vi "ActionVIOnCompile.vi"(8 "error in (no error)":errorcluster, 11 "Device Item Ref in":T1 format="%.0x") -> (0 "error out":errorcluster)   [LabVIEW 2024, in "Nominal Client System Explorer.lvlib"]
uses:
  Nominal Client System Explorer.lvlib
  <vilib>/NI VeriStand/Custom Device API/Custom Device Item Ref.ctl
  Shared/Compiled.Settings.ctl
  <vilib>/NI VeriStand/Custom Device API/Get Item Property (U16).vi
  <vilib>/NI VeriStand/Custom Device API/Set Item Property (Variant).vi
  <vilib>/NI VeriStand/Custom Device Tools/Custom Device Utility Library/Custom Device Utility Library.lvlib
  <vilib>/NI VeriStand/Custom Device Tools/Custom Device Utility Library/NI VeriStand - Search for Item by Name.vi
  <vilib>/NI VeriStand/Custom Device API/Custom Device API.lvlib
  <vilib>/NI/NIVS Inline Async API/_Data Access System Explorer/Data Access System Explorer.lvlib
  Shared/Nominal Client Shared.lvlib
  Scripting/Nominal Client Scripting.lvlib
  Built/Nominal Client/Windows/nominal-labview-client.lvlibp
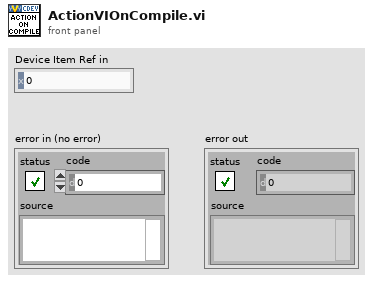
[diagram p1: front panel]
types:
  T1 = typedef "Custom Device API.lvlib/Custom Device Item Ref.ctl" = u64
  T2 = cluster{"Name":string, "Type":enum16{"Output/Write", "Input/Read", "Input/ReadWrite"}, "VS Refs":T1[]}
  T3 = enum16{"Output/Write", "Input/Read", "Input/ReadWrite"}
  T4 = enum16{"open", "replace", "create", "open or create", "replace or create", "replace or create with confirmation"}
  T5 = typedef "Nominal Client Shared.lvlib/Compiled.Settings.ctl" = cluster{"Name":string, "Async Init Timeout":u16, "api key":string}
  T6 = typedef "Custom Device API.lvlib/Custom Device Item Info.ctl" = cluster{"Name":string, "Is Channel":bool, "GUID":string, "Is Waveform":bool}
  T7 = cluster{"Name":string, "Type":enum16{"Output/Write", "Input/Read", "Input/ReadWrite"}, "VS Refs":T1[]}[]
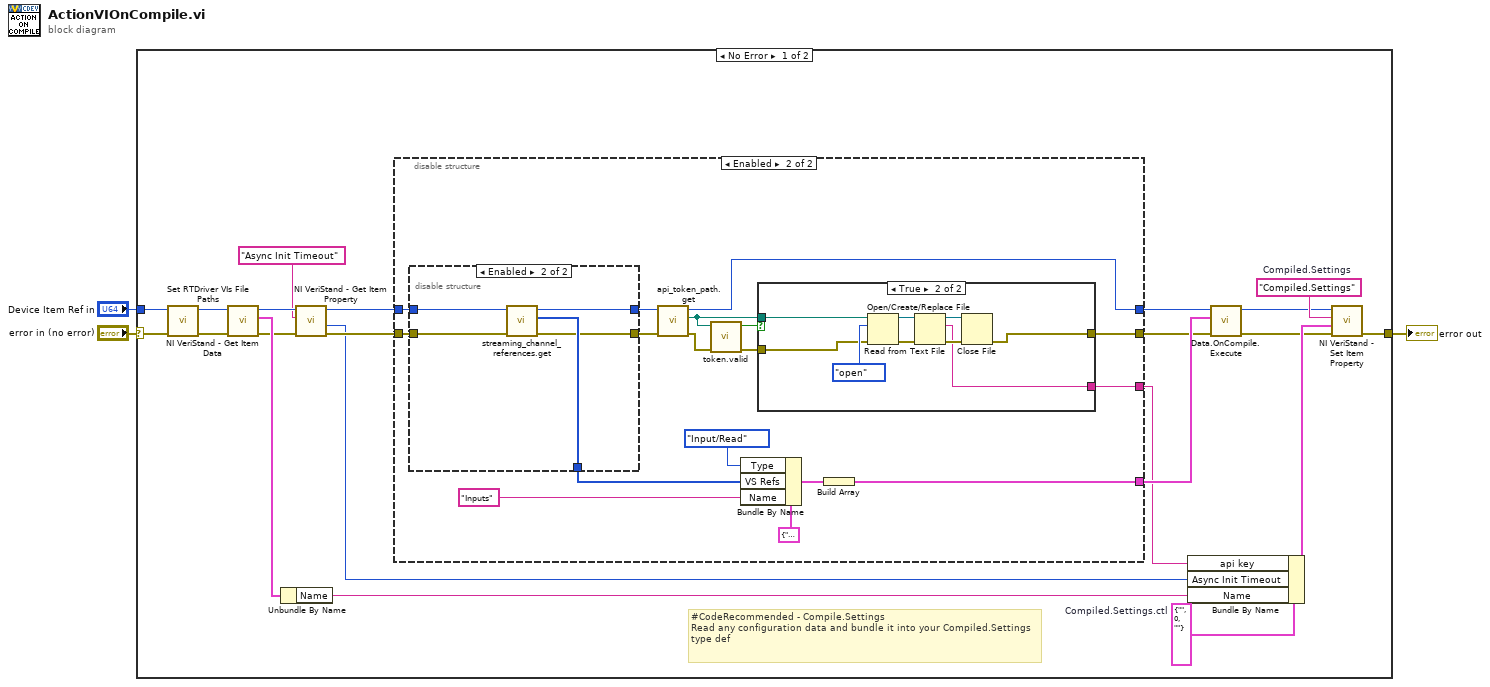
[diagram p0: block diagram]
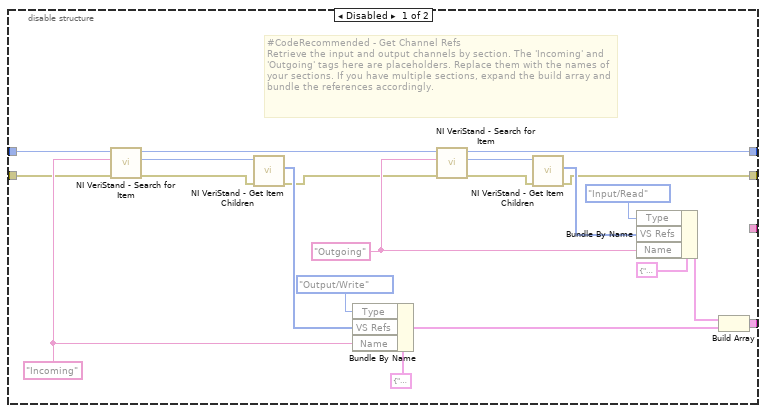
[diagram p2: hidden frame]
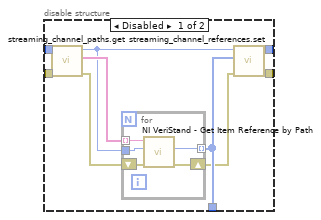
[diagram p3: hidden frame]
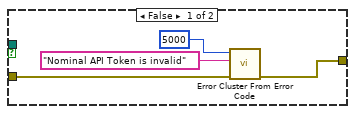
[diagram p4: hidden frame]
diagram:
  n1 = case shown="No Error" "error in (no error)" {
    selector: "error in (no error)" -> [w7 w96]
    tunnel: [w23 w96] -> w2
    tunnel: "Device Item Ref in" -> [w8 _]
    frame No Error {
      w15 = T5 {"Name"="", "Async Init Timeout"=0, "api key"=""}  # Compiled.Settings.ctl
      w25 = "Compiled.Settings"  # Compiled.Settings
      # "#CodeRecommended - Compile.Settings\nRead any configuration data and bundle it into your Compiled.Settings type def"
      n2 = call "Set RTDriver VIs File Paths.vi"("error in (no error)"=w7, "Item Ref in"=w8) -> ("error out"=w5:errorcluster, "Item Ref out"=w6:T1)  [unwired: 8 in]
      n3 = call <vilib>:"NI VeriStand - Get Item Data.vi"("error in (no error)"=w5, "Item Ref in"=w6) -> ("error out"=w14:errorcluster, "Item Info"=w22:T6, "Item Ref out"=w12:T1)  [unwired: 6 in, 1 out]
      n4 = Unbundle By Name(w22) -> ("Name"=w21:string)
      n5 = call-poly <vilib>:"NI VeriStand - Get Item Property.vi"("error in (no error)"=w14, "Property Name"="Async Init Timeout", "Item Ref in"=w12) -> ("error out"=w13:errorcluster, "Value"=w9:u16, "Item Ref out"=w11:T1)  [unwired: 5 in, 1 out]
      n6 = disable-structure shown="Enabled" {
        disable-tunnel: [w37 w59] -> w20
        disable-tunnel: [w33 w57] -> w19
        disable-tunnel: [w32 w58] -> w18
        disable-tunnel: w13 -> [w29 w50]
        disable-tunnel: w11 -> [w28 w51]
        disable-tunnel: [_ w56] -> w4
        frame Disabled {
          w42 = "Outgoing" ("Item Name")
          w44 = "Incoming" ("Item Name")
          # "#CodeRecommended - Get Channel Refs\nRetrieve the input and output channels by section. The 'Incoming' and 'Outgoing' tags here are placeholders. Replace them with the names of your sections. If you have multiple sections, expand the build array and bundle the references accordingly."
          n7 = call-poly <vilib>:"NI VeriStand - Search for Item.vi"("error in"=w29, "Item Name"=w44, "Section Ref in"=w28) -> ("error out"=w27:errorcluster, "Item Ref"=w26:T1, "Section Ref out"=w31:T1)  [unwired: 5 in, 1 out]
          n8 = call <vilib>:"NI VeriStand - Get Item Children.vi"("error in (no error)"=w27, "Item Ref in"=w26) -> ("error out"=w30:errorcluster, "Child Refs"=w43:T1[])  [unwired: 6 in, 2 out]
          n9 = Bundle By Name(cluster=T2 {"Name"="", "Type"=enum."Output/Write", "VS Refs"=[]} ("Group"), "Type"=T3."Output/Write", "VS Refs"=w43, "Name"=w44) -> (w34:T2)
          n10 = call-poly <vilib>:"NI VeriStand - Search for Item.vi"("error in"=w30, "Item Name"=w42, "Section Ref in"=w31) -> ("error out"=w45:errorcluster, "Item Ref"=w46:T1, "Section Ref out"=w32:T1)  [unwired: 5 in, 1 out]
          n11 = call <vilib>:"NI VeriStand - Get Item Children.vi"("error in (no error)"=w45, "Item Ref in"=w46) -> ("error out"=w33:errorcluster, "Child Refs"=w38:T1[])  [unwired: 6 in, 2 out]
          n12 = Bundle By Name(cluster=T2 {"Name"="", "Type"=enum."Output/Write", "VS Refs"=[]} ("Group"), "Type"=T3."Input/Read", "VS Refs"=w38, "Name"=w42) -> (w40:T2)
          n13 = Build Array(w40, w34) -> (w37:T7)
        }
        frame Enabled {
          n14 = disable-structure shown="Enabled" {
            disable-tunnel: w51 -> [w71 w82]
            disable-tunnel: w50 -> [w70 w78]
            disable-tunnel: [w69 w80] -> w49
            disable-tunnel: [w68 w79] -> w48
            disable-tunnel: [w67 w81] -> w47
            frame Disabled {
              n15 = call "streaming_channel_paths.get.vi"("error in (no error)"=w70, "Item Ref in"=w71) -> ("error out"=w65:errorcluster, "Channel Paths"=w72:string[], "Item Ref out"=w66:T1)  [unwired: 7 in]
              n16 = for {
                tunnel: w72 -> [w77] mode=indexing
                tunnel: [w76] -> w67 mode=indexing
                tunnel: w66 -> [w75]
                shift-right: [w74] -> w64
                shift-left: w65 -> [w73]
                n17 = call <vilib>:"NI VeriStand - Get Item Reference by Path.vi"("error in (no error)"=w73, "Root Ref"=w75, "Item Path in"=w77) -> ("error out"=w74:errorcluster, "Item Ref"=w76:T1)  [unwired: 5 in, 2 out]
              }
              n18 = call "streaming_channel_references.set.vi"("error in (no error)"=w64, "Dependent Node Refs"=w67, "Item Ref in"=w66) -> ("error out"=w68:errorcluster, "Item Ref out"=w69:T1)  [unwired: 7 in]
            }
            frame Enabled {
              n19 = call "streaming_channel_references.get.vi"("error in (no error)"=w78, "Item Ref in"=w82) -> ("error out"=w79:errorcluster, "Streaming Channel Refs"=w81:T1[], "Item Ref out"=w80:T1)  [unwired: 7 in]
            }
          }
          n20 = call "api_token_path.get.vi"("error in (no error)"=w48, "Nominal IO Client in"=w49) -> ("error out"=w54:errorcluster, "API Token file"=w55:path, "Nominal IO Client out"=w58:T1)  [unwired: 6 in, 1 out]
          n21 = call "token.valid.vi"("error in"=w54, "token"=w55) -> ("error out"=w53:errorcluster, "valid"=w52:bool)  [unwired: 8 in]
          n22 = Bundle By Name(cluster=T2 {"Name"="", "Type"=enum."Output/Write", "VS Refs"=[]} ("Group"), "Type"=T3."Input/Read", "VS Refs"=w47, "Name"="Inputs") -> (w60:T2)
          n23 = case shown="True" w52 {
            tunnel: [w83 w90] -> w57
            tunnel: [_ w89] -> w56
            tunnel: w55 -> [_ w88]
            tunnel: w53 -> [w84 w87]
            frame False {
              n24 = call <vilib>:"Error Cluster From Error Code.vi"("error in (no error)"=w84, "error message (\"\")"="Nominal API Token is invalid" ("error message (\"\")"), "error code (0)"=5000) -> ("error out"=w83:errorcluster)  [unwired: 6 in]
            }
            frame True {
              n25 = Open/Create/Replace File(file path (use dialog)=w88, error in=w87, operation (0:open)=T4."open") -> (refnum out=w94:refnum<file>, error out=w92:errorcluster)  [unwired: 3 in, 1 out]
              n26 = Read from Text File(file (use dialog)=w94, error in=w92) -> (refnum out=w95:refnum<file>, text=w89:string, error out=w93:errorcluster)  [unwired: 2 in, 1 out]
              n27 = Close File(refnum=w95, error in=w93) -> (error out=w90:errorcluster)  [unwired: 1 out]
            }
          }
          n28 = Build Array(w60) -> (w59:T7)
        }
      }
      n29 = Bundle By Name(cluster=w15, "api key"=w4, "Async Init Timeout"=w9, "Name"=w21) -> (w24:T5)
      n30 = call <vilib>:"Data.OnCompile.Execute.vi"("error in"=w19, "VS Ref Groups"=w20, "Custom Device Ref"=w18) -> ("error out"=w17:errorcluster, "Custom Device Ref"=w16:T1)  [unwired: 7 in]
      n31 = call-poly <vilib>:"NI VeriStand - Set Item Property.vi"("error in (no error)"=w17, "Value"=w24, "Property Name"=w25, "Item Ref in"=w16) -> ("error out"=w23:errorcluster)  [unwired: 5 in, 2 out]
    }
    frame Error {
    }
  }
  "error out" <- w2
